vi "RecongnizedResult.vi"(4 "SR_REC_TEXT":refnum<vi>, 5 "事件数据":cluster{"sender":refnum<k24>, "e":refnum<k24>}, 6 "控件引用":refnum<k24>, 7 "事件通用数据":cluster{"事件源":i32, "事件类型":u32, "时间标识":u32}) -> ()   [LabVIEW 2018]
uses:
  System.Speech
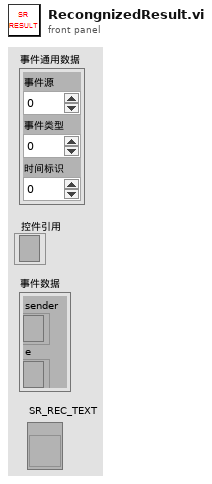
[diagram p1: front panel]
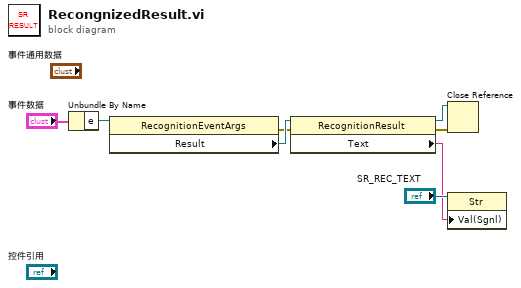
[diagram p0: block diagram]
diagram:
  n1 = Unbundle By Name("事件数据") -> ("e"=w7:refnum<k24>)
  n2 = property class="RecognitionEventArgs"(reference=w7) -> (error out=w4:errorcluster, "Result"=w6:refnum<k24>)  [unwired: 1 in, 1 out]
  n3 = property class="RecognitionResult"(reference=w6, error in=w4) -> (reference out=w5:refnum<k24>, error out=w3:errorcluster, "Text"=w1:string)
  n4 = Close Reference(reference=w5, error in (no error)=w3) -> ()  [unwired: 1 out]
  n5 = property class="Str"(reference="SR_REC_TEXT", "Val(Sgnl)"=w1) -> ()  [unwired: 1 in, 2 out]
